vi "local_veriable_racing.vi"() -> ()   [LabVIEW 2021]
uses:
  119b6580-82b5-3fb2-b6d0-fd24739be03f.vi
  995ef0fa-1257-3fef-196f-f408f134e23f.vi
panel:
  in  "Numeric":i32
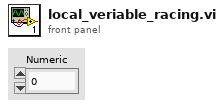
[diagram p1: front panel]
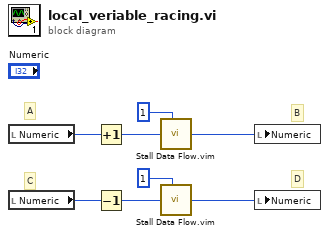
[diagram p0: block diagram]
diagram:
  # "D"
  # "C"
  # "B"
  # "A"
  n1 = local read "Numeric"() -> (w7:i32)
  n2 = local read "Numeric"() -> (w8:i32)
  n3 = Increment(x=w7) -> (x+1=w6:i32)
  n4 = Decrement(x=w8) -> (x-1=w3:i32)
  n5 = call "Stall Data Flow.vim"("value in"=w6, "milliseconds to wait"=u32 1) -> ("value out"=w5:i32)  [unwired: 1 out]
  n6 = call "Stall Data Flow.vim"("value in"=w3, "milliseconds to wait"=u32 1) -> ("value out"=w2:i32)  [unwired: 1 out]
  n7 = local write "Numeric"(w5) -> ()
  n8 = local write "Numeric"(w2) -> ()
